vi "Test Harness.vi"() -> ()   [LabVIEW 2015, in "Waveform-Processing-Custom-Device Engine.lvlib"]
uses:
  Waveform-Processing-Custom-Device Engine.lvlib
  <vilib>/NI Veristand/Custom Device API/Hardware Interface Driver VI Operation.ctl
  <vilib>/NI Veristand/Custom Device API/Custom Device Item Ref.ctl
  <vilib>/NI VeriStand/Custom Device API/Custom Device API.lvlib
  <vilib>/Analysis/NI_AALBase.lvlib
panel:
  in  "Wfm Gen Loop Count":u32=25
  out "size(s)":i32[](array[numeric])
  in  "amplitude":dbl=1.0 format="%0.2f"
  in  "Number of Waveforms":i32=2
  in  "Loop Rate":u32=100
  in  "Stop":bool
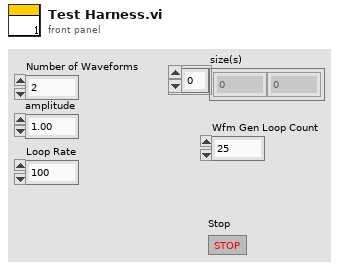
[diagram p1: front panel]
types:
  T1 = typedef "Custom Device API.lvlib/Hardware Interface Driver VI Operation.ctl" = enum16{"Initialize", "Start", "Read Data from HW", "Write Data to HW", "Close"}
  T2 = typedef "Custom Device API.lvlib/Custom Device Item Ref.ctl" = u64
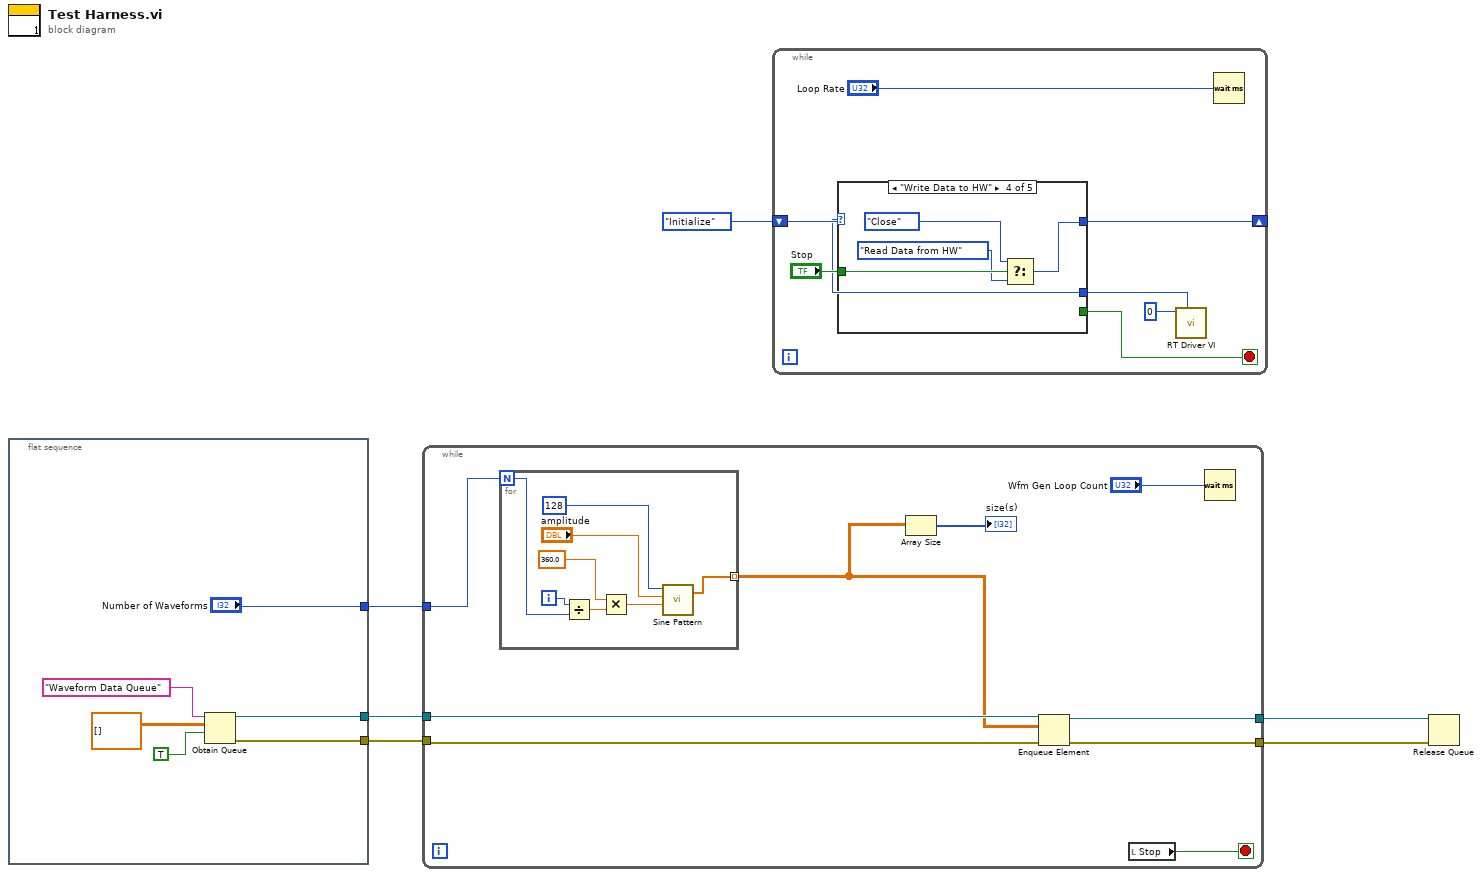
[diagram p0: block diagram]
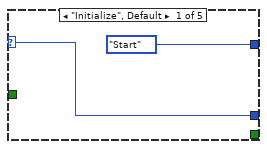
[diagram p2: hidden frame]
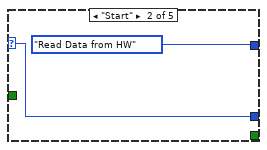
[diagram p3: hidden frame]
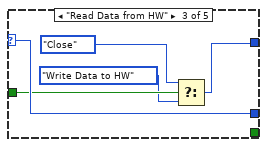
[diagram p4: hidden frame]
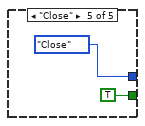
[diagram p5: hidden frame]
diagram:
  n1 = flat-sequence {
    tunnel: [w9] -> w4
    tunnel: [w8] -> w5
    tunnel: ["Number of Waveforms"] -> w1
    frame #0 {
      n2 = Obtain Queue(name (unnamed)="Waveform Data Queue", element data type=dbl[][] [], create if not found? (T)=TRUE) -> (queue out=w8:refnum<queue>, error out=w9:errorcluster)  [unwired: 2 in, 1 out]
    }
  }
  n3 = while {
    tunnel: w5 -> [w17]
    tunnel: w4 -> [w16]
    tunnel: [w20] -> w3
    tunnel: [w19] -> w2
    tunnel: w1 -> [w18]
    stop <- w21 stop-if-true
    n4 = for {
      N: w18 -> [w28]
      tunnel: [w23] -> w15 mode=indexing
      i -> [w29]
      n5 = Divide(x=w29, y=w28) -> (x/y=w27:dbl)
      n6 = Multiply(x=360.0, y=w27) -> (x*y=w25:dbl)
      n7 = call <vilib>:"Sine Pattern.vi"("phase(degrees)"=w25, "amplitude"="amplitude", "samples"=128) -> ("Sinusoidal Pattern"=w23:dbl[])  [unwired: 1 in, 1 out]
    }
    n8 = Array Size(array=w15) -> (size(s)=→"size(s)":i32[])
    n9 = Enqueue Element(queue=w17, element=w15, error in (no error)=w16) -> (queue out=w19:refnum<queue>, error out=w20:errorcluster)  [unwired: 1 in, 1 out]
    n10 = local read "Stop"() -> (w21:bool)
    n11 = Wait (ms)(milliseconds to wait="Wfm Gen Loop Count") -> ()  [unwired: 1 out]
  }
  n12 = while {
    shift-right: [w34] -> _
    shift-left: Hardware_Interface_Driver_VI_Operation."Initialize" ("Operation") -> [w36]
    stop <- w32 stop-if-true
    n13 = case shown="\"Write Data to HW\"" w36 {
      selector: w36 -> [w38 w39 w45 w50 _]
      tunnel: [w38 w39 w45 w50 Hardware_Interface_Driver_VI_Operation."Close" ("Operation")] -> w35
      tunnel: [Hardware_Interface_Driver_VI_Operation."Start" ("Operation") Hardware_Interface_Driver_VI_Operation."Read Data from HW" ("Operation") w41 w46 _] -> w34
      tunnel: "Stop" -> [_ _ w44 w49 _]
      tunnel: [_ _ _ _ TRUE] -> w32
      frame "Initialize", Default {
      }
      frame "Start" {
      }
      frame "Read Data from HW" {
        n14 = Select(t=Hardware_Interface_Driver_VI_Operation."Close" ("Operation"), s=w44, f=Hardware_Interface_Driver_VI_Operation."Write Data to HW" ("Operation")) -> (s? t:f=w41:T1)
      }
      frame "Write Data to HW" {
        n15 = Select(t=Hardware_Interface_Driver_VI_Operation."Close" ("Operation"), s=w49, f=Hardware_Interface_Driver_VI_Operation."Read Data from HW" ("Operation")) -> (s? t:f=w46:T1)
      }
      frame "Close" {
      }
    }
    n16 = call "RT Driver VI.vi"("Operation"=w35, "Device Reference in"=T2 0) -> ()  [unwired: 9 in, 1 out]
    n17 = Wait (ms)(milliseconds to wait="Loop Rate") -> ()  [unwired: 1 out]
  }
  n18 = Release Queue(queue=w2, error in (no error)=w3) -> ()  [unwired: 1 in, 3 out]
